vi "Tell Child.vi"(4 "Priority":bool, 6 "UID":string, 10 "Msg":refnum<class "Msg.lvclass">, 11 "Core Actor in":refnum<class "Core Actor.lvclass">) -> (0 "Error out":errorcluster)   [LabVIEW 2025, in "jettl.lvlib" / "Actor.lvlib" / "Core Actor.lvclass"]
uses:
  Core Actor.lvclass
  Msg/Msg.lvclass
  Relation.ctl
  Attributes/Attributes/Attributes.lvclass
  Transport/Transport/Transport.lvclass
  Core Actor.lvclass/Core Actor.ctl
  jettl.lvlib
  Error/Error.lvlib
  Actor.lvlib
  Teller/Teller.lvlib
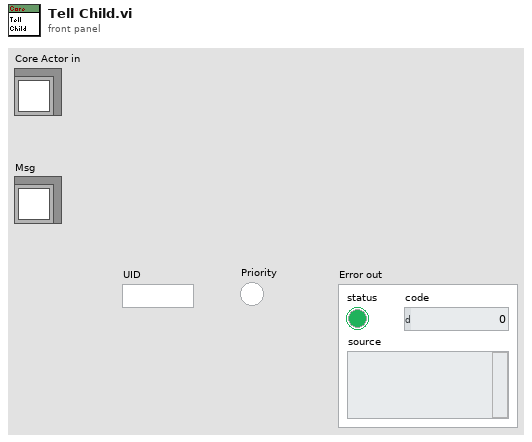
[diagram p1: front panel]
types:
  T1 = typedef "jettl.lvlib/Actor.lvlib/Relation.ctl" = enum16{"Self", "Parent", "Child"}
  T2 = typedef "jettl.lvlib/Actor.lvlib/Msg Set.ctl" = set{refnum<class "Msg.lvclass">}
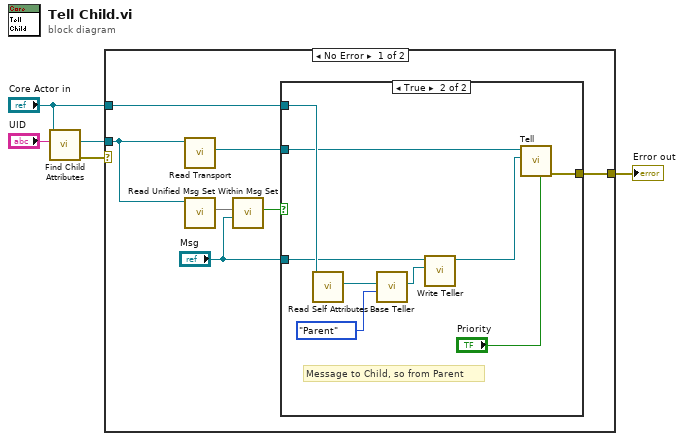
[diagram p0: block diagram]
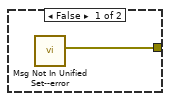
[diagram p2: hidden frame]
diagram:
  n1 = call-dynamic "Find Child Attributes.vi"("UID"="UID", "Core Actor in"="Core Actor in") -> ("Error out"=w2:errorcluster, "Child Attributes"=w1:refnum<class "Attributes.lvclass">)  [unwired: 8 in]
  n2 = case shown="No Error" w2 {
    selector: w2 -> [_ w23]
    tunnel: "Core Actor in" -> [w7 _]
    tunnel: [w12 w23] -> w5
    tunnel: w1 -> [w6 _]
    frame No Error {
      n3 = call-dynamic "Read Transport.vi"("Attributes in"=w6) -> ("Transport"=w9:refnum<class "Transport.lvclass">)  [unwired: 10 in]
      n4 = call-dynamic "Read Unified Msg Set.vi"("Attributes in"=w6) -> ("Unified Msg Set"=w11:T2)  [unwired: 10 in]
      n5 = call "Within Msg Set.vi"("Msg"="Msg", "Msg Set"=w11) -> ("Within Msg Set"=w10:bool)  [unwired: 9 in]
      n6 = case shown="True" w10 {
        tunnel: w7 -> [_ w22]
        tunnel: "Msg" -> [_ w20]
        tunnel: [w13 w14] -> w12
        tunnel: w9 -> [_ w17]
        frame False {
          n7 = call "Msg Not In Unified Set--error.vi"() -> ("Error"=w13:errorcluster)  [unwired: 11 in]
        }
        frame True {
          # "Message to Child, so from Parent"
          n8 = call-dynamic "Read Self Attributes.vi"("Core Actor in"=w22) -> ("Self Attributes"=w18:refnum<class "Attributes.lvclass">)  [unwired: 10 in]
          n9 = call "Base Teller.vi"("Relation"=Relation."Parent", "Self Attributes"=w18) -> ("Teller"=w21:refnum<class "Teller.lvclass">)  [unwired: 9 in]
          n10 = call-dynamic "Write Teller.vi"("Teller"=w21, "Msg in"=w20) -> ("Msg out"=w16:refnum<class "Msg.lvclass">)  [unwired: 9 in]
          n11 = call-dynamic "Tell.vi"("Priority"="Priority", "Msg"=w16, "Transport in"=w17) -> ("Error out"=w14:errorcluster)  [unwired: 8 in]
        }
      }
    }
    frame Error {
    }
  }
  "Error out" <- w5
